vi "sub_main_joystick.vi"(8 "error in":errorcluster) -> (0 "error out":errorcluster)   [LabVIEW 2019]
uses:
  Ctrl/cmd_common.ctl
  Ctrl/sound-data.ctl
panel:
  out "error out check":errorcluster
  out "n":i32
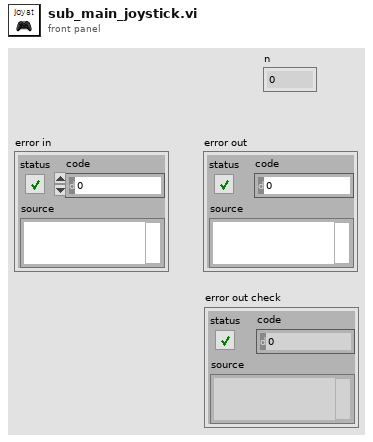
[diagram p1: front panel]
types:
  T1 = typedef "cmd_common.ctl" = enum16{"read", "write"}
  T2 = typedef "sound-data.ctl" = cluster{"FN":enum16{"check", "unlock", "engine", "warning", "msg", "music"}, "Data":variant}
  T3 = cluster{"axis info":cluster{"X axis":i32, "Y axis":i32, "Z axis":i32, "X axis rotation":i32, "Y axis rotation":i32, "Z axis rotation":i32, "U axis":i32, "V axis":i32}, "button info":cluster{"button 1":bool, "button 2":bool, "button 3":bool, "button 4":bool, "button 5":bool, "button 6":bool, "button 7":bool, "button 8":bool, "button 9":bool, "button 10":bool, "button 11":bool, "button 12":bool, "button 13":bool, "button 14":bool, "button 15":bool, "button 16":bool, "button 17":bool, "button 18":bool, "button 19":bool, "button 20":bool, "button 21":bool, "button 22":bool, "button 23":bool, "button 24":bool, "button 25":bool, "button 26":bool, "button 27":bool, "button 28":bool, "button 29":bool, "button 30":bool, "button 31":bool, "button 32":bool}, "direction info":cluster{"pov 1":i32, "pov 2":i32, "pov 3":i32, "pov 4":i32}}
  T4 = cluster{"button 1":bool, "button 2":bool, "button 3":bool, "button 4":bool, "button 5":bool, "button 6":bool, "button 7":bool, "button 8":bool, "button 9":bool, "button 10":bool, "button 11":bool, "button 12":bool, "button 13":bool, "button 14":bool, "button 15":bool, "button 16":bool, "button 17":bool, "button 18":bool, "button 19":bool, "button 20":bool, "button 21":bool, "button 22":bool, "button 23":bool, "button 24":bool, "button 25":bool, "button 26":bool, "button 27":bool, "button 28":bool, "button 29":bool, "button 30":bool, "button 31":bool, "button 32":bool}
  T5 = cluster{"pov 1":i32, "pov 2":i32, "pov 3":i32, "pov 4":i32}
  T6 = enum16{"check", "unlock", "engine", "warning", "msg", "music"}
  T7 = typedef "status.ctl" = u16
  T8 = cluster{"AGV":T7, "AGV Estop":T7, "Obstacle":T7, "Heading":T7, "Waypt":T7, "GNSS":T7, "VLP16":T7, "Cam":T7, "RPLidar":T7, "Joystick":T7, "IMU":T7}
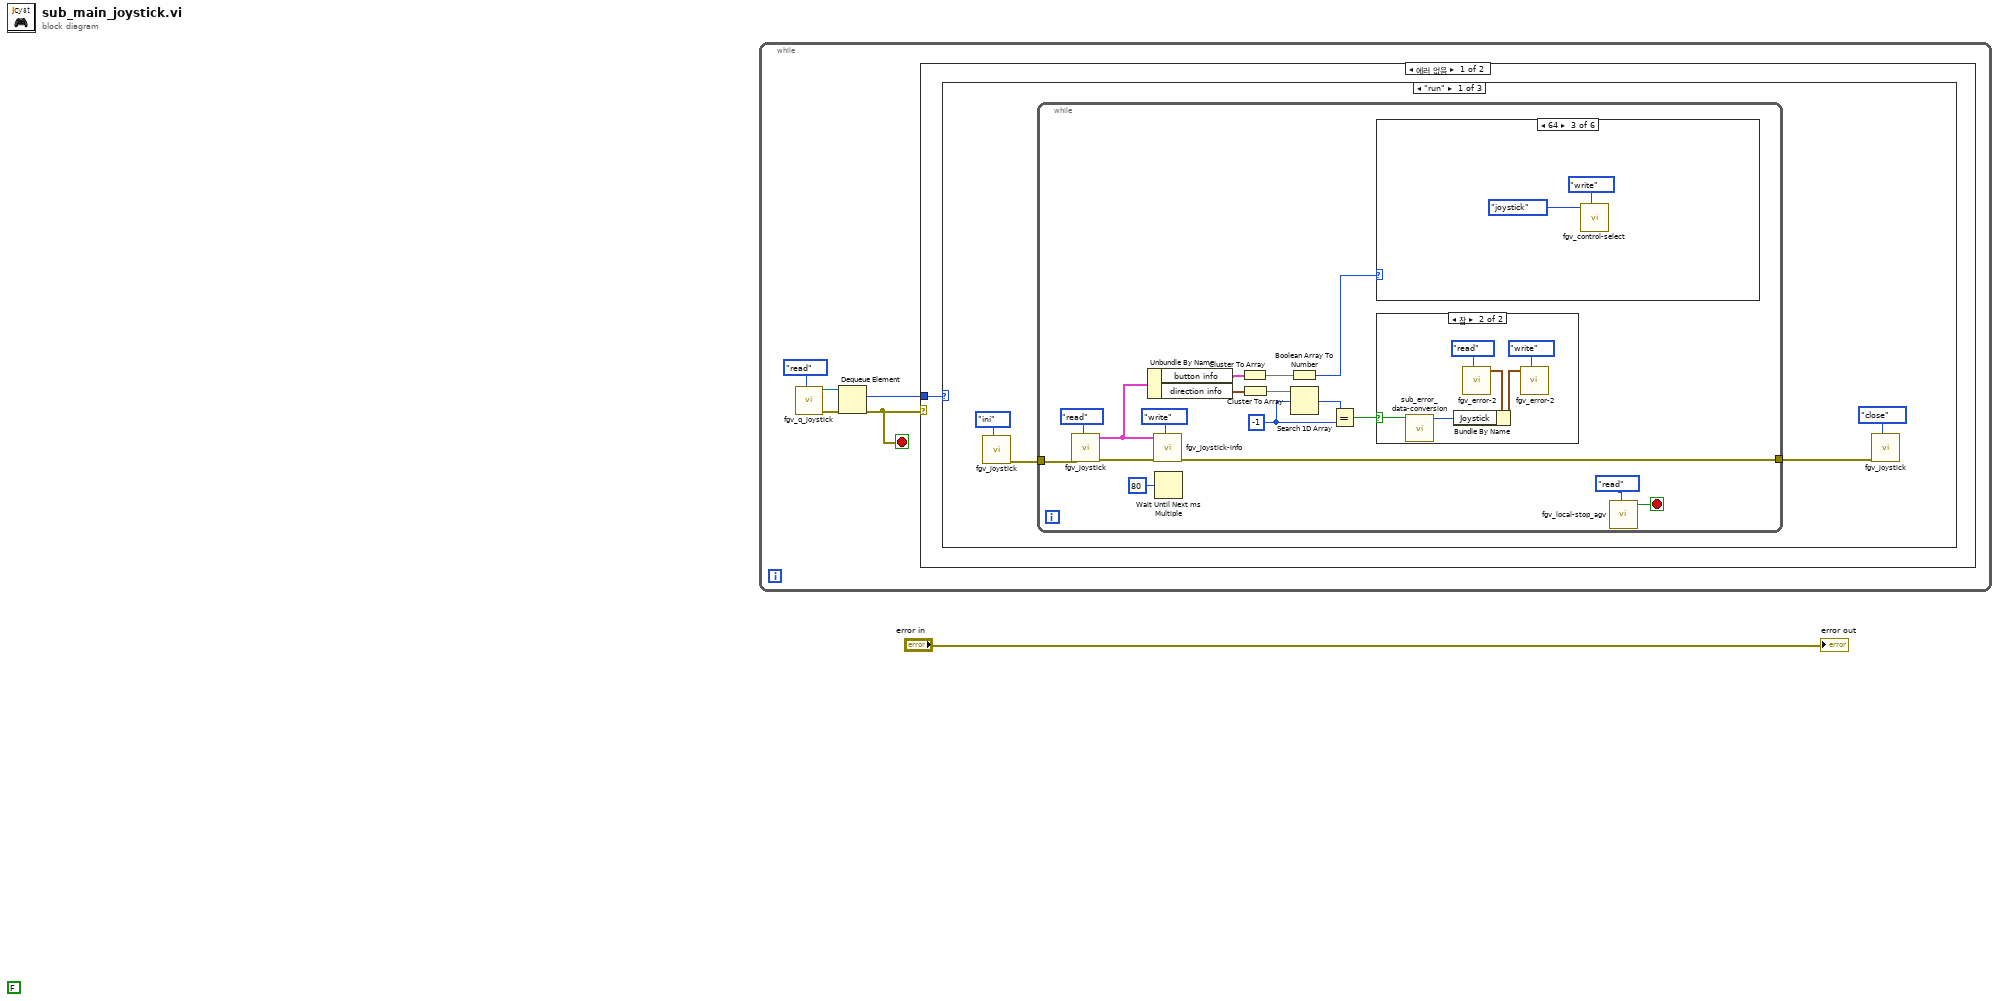
[diagram p0: block diagram]
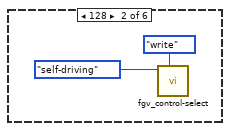
[diagram p3: hidden frame]
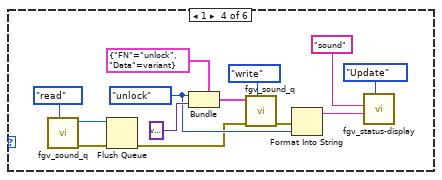
[diagram p4: hidden frame]
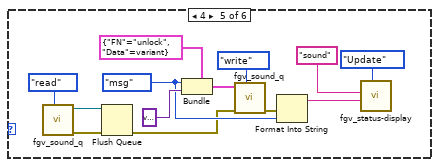
[diagram p5: hidden frame]
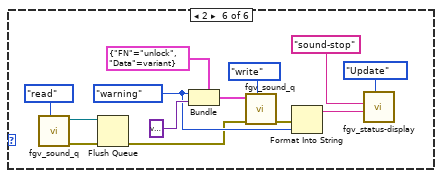
[diagram p6: hidden frame]
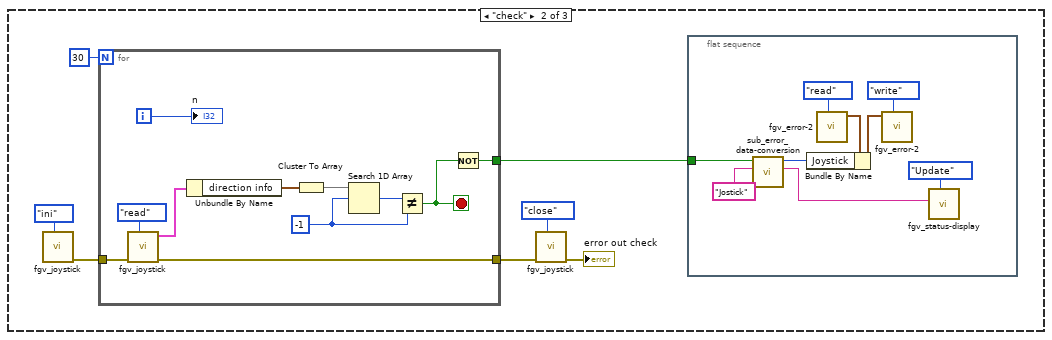
[diagram p8: hidden frame]
diagram:
  (unwired) FALSE
  n1 = while {
    stop <- w2 stop-if-true
    n2 = call "fgv_q_joystick.vi"("cmd"=enum16{"create", "write", "read", "close"}."read") -> ("error out"=w4:errorcluster, "queue out"=w5:refnum<queue>)  [unwired: 9 in]
    n3 = Dequeue Element(queue=w5, error in (no error)=w4) -> (element=w3:enum16{"run", "check", "stop"}, error out=w2:errorcluster)  [unwired: 1 in, 2 out]
    n4 = case shown="에러 없음" w2 {
      tunnel: w3 -> [w7 _]
      frame No Error {
        n5 = case shown="\"run\"" w7 {
          frame "run" {
            n6 = call "fgv_joystick.vi"("cmd"=enum16{"ini", "read", "close"}."ini") -> ("error out"=w9:errorcluster)  [unwired: 9 in, 1 out]
            n7 = while {
              tunnel: w9 -> [w23]
              tunnel: [w22] -> w8
              stop <- w27 stop-if-true
              w18 = -1 ("element")
              n8 = call "fgv_joystick.vi"("cmd"=enum16{"ini", "read", "close"}."read", "error in"=w23) -> ("error out"=w24:errorcluster, "joystick info-out"=w17:T3)  [unwired: 8 in]
              n9 = Unbundle By Name(w17) -> ("button info"=w14:T4, "direction info"=w21:T5)
              n10 = call "fgv_joystick-info.vi"("init"=enum16{"enable", "init", "read", "write"}."write", "error in"=w24, "joystick info-in"=w17) -> ("error out"=w22:errorcluster)  [unwired: 5 in, 3 out]
              n11 = Wait Until Next ms Multiple(millisecond multiple=u32 80 ("milliseconds to wait")) -> ()  [unwired: 1 out]
              n12 = Cluster To Array(cluster=w14) -> (array=w13:bool[])
              n13 = Cluster To Array(cluster=w21) -> (array=w20:i32[])
              n14 = Boolean Array To Number(Boolean array=w13) -> (number=w12:u32)
              n15 = Search 1D Array(1D array=w20, element=w18) -> (index of element=w19:i32)  [unwired: 1 in]
              n16 = Equal?(x=w19, y=w18) -> (x = y?=w15:bool)
              n17 = case shown="64" w12 {
                frame 0, Default {
                }
                frame 128 {
                  n18 = call "fgv_control-select.vi"("cmd"=cmd_common."write", "mode"=enum16{"joystick", "self-driving"}."self-driving") -> ()  [unwired: 9 in, 1 out]
                }
                frame 64 {
                  n19 = call "fgv_control-select.vi"("cmd"=cmd_common."write", "mode"=enum16{"joystick", "self-driving"}."joystick") -> ()  [unwired: 9 in, 1 out]
                }
                frame 1 {
                  w38 = T6."unlock" ("FN")
                  n20 = call "fgv_sound_q.vi"("cmd"=enum16{"create", "write", "read", "close"}."read") -> ("error out"=w35:errorcluster, "queue out"=w34:refnum<queue>)  [unwired: 9 in]
                  n21 = Flush Queue(queue=w34, error in (no error)=w35) -> (error out=w33:errorcluster)  [unwired: 2 out]
                  n22 = Bundle(cluster=T2 {"FN"=enum."unlock", "Data"=variant} ("data"), "FN"=w38, "Data"=variant) -> (w44:T2)
                  n23 = call "fgv_sound_q.vi"("cmd"=enum16{"create", "write", "read", "close"}."write", "error in"=w33, "data"=w44) -> ("error out"=w39:errorcluster)  [unwired: 7 in, 1 out]
                  n24 = Format Into String(error in=w39, w38) -> (resulting string=w37:string)  [unwired: 2 in, 1 out]
                  n25 = call "fgv_status-display.vi"("Mode"=enum16{"Initial", "Update", "Clear"}."Update", "detail"=w37, "title"="sound") -> ()  [unwired: 8 in, 1 out]
                }
                frame 4 {
                  w51 = T6."msg" ("FN")
                  n26 = call "fgv_sound_q.vi"("cmd"=enum16{"create", "write", "read", "close"}."read") -> ("error out"=w48:errorcluster, "queue out"=w47:refnum<queue>)  [unwired: 9 in]
                  n27 = Flush Queue(queue=w47, error in (no error)=w48) -> (error out=w46:errorcluster)  [unwired: 2 out]
                  n28 = Bundle(cluster=T2 {"FN"=enum."unlock", "Data"=variant} ("data"), "FN"=w51, "Data"=variant) -> (w57:T2)
                  n29 = call "fgv_sound_q.vi"("cmd"=enum16{"create", "write", "read", "close"}."write", "error in"=w46, "data"=w57) -> ("error out"=w52:errorcluster)  [unwired: 7 in, 1 out]
                  n30 = Format Into String(error in=w52, w51) -> (resulting string=w50:string)  [unwired: 2 in, 1 out]
                  n31 = call "fgv_status-display.vi"("Mode"=enum16{"Initial", "Update", "Clear"}."Update", "detail"=w50, "title"="sound") -> ()  [unwired: 8 in, 1 out]
                }
                frame 2 {
                  w64 = T6."warning" ("FN")
                  n32 = call "fgv_sound_q.vi"("cmd"=enum16{"create", "write", "read", "close"}."read") -> ("error out"=w61:errorcluster, "queue out"=w60:refnum<queue>)  [unwired: 9 in]
                  n33 = Flush Queue(queue=w60, error in (no error)=w61) -> (error out=w59:errorcluster)  [unwired: 2 out]
                  n34 = Bundle(cluster=T2 {"FN"=enum."unlock", "Data"=variant} ("data"), "FN"=w64, "Data"=variant) -> (w70:T2)
                  n35 = call "fgv_sound_q.vi"("cmd"=enum16{"create", "write", "read", "close"}."write", "error in"=w59, "data"=w70) -> ("error out"=w65:errorcluster)  [unwired: 7 in, 1 out]
                  n36 = Format Into String(error in=w65, w64) -> (resulting string=w63:string)  [unwired: 2 in, 1 out]
                  n37 = call "fgv_status-display.vi"("Mode"=enum16{"Initial", "Update", "Clear"}."Update", "detail"=w63, "title"="sound-stop") -> ()  [unwired: 8 in, 1 out]
                }
              }
              n38 = case shown="참" w15 {
                selector: w15 -> [_ w72]
                frame False {
                }
                frame True {
                  n39 = call "sub_error_data-conversion.vi"("error status"=w72) -> ("error conversion out"=w75:T7)  [unwired: 9 in, 1 out]
                  n40 = call "fgv_error-2.vi"("cmd"=enum16{"init", "read", "write"}."read") -> ("Error cluster out"=w74:T8)  [unwired: 9 in, 1 out]
                  n41 = Bundle By Name(cluster=w74, "Joystick"=w75) -> (w73:T8)
                  n42 = call "fgv_error-2.vi"("cmd"=enum16{"init", "read", "write"}."write", "Error cluster"=w73) -> ()  [unwired: 8 in, 2 out]
                }
              }
              n43 = call "fgv_local-stop_agv.vi"("cmd"=enum16{"ini", "read", "stop"}."read") -> ("stop status"=w27:bool)  [unwired: 10 in]
            }
            n44 = call "fgv_joystick.vi"("cmd"=enum16{"ini", "read", "close"}."close", "error in"=w8) -> ()  [unwired: 8 in, 2 out]
          }
          frame "check" {
            n45 = call "fgv_joystick.vi"("cmd"=enum16{"ini", "read", "close"}."ini") -> ("error out"=w83:errorcluster)  [unwired: 9 in, 1 out]
            n46 = for {
              N: 30 -> [_]
              tunnel: w83 -> [w104]
              tunnel: [w96] -> w80
              tunnel: [w94] -> w78
              i -> [w97]
              stop <- w95 stop-if-true
              w102 = -1 ("element")
              n47 = call "fgv_joystick.vi"("cmd"=enum16{"ini", "read", "close"}."read", "error in"=w104) -> ("error out"=w96:errorcluster, "joystick info-out"=w98:T3)  [unwired: 8 in]
              n48 = Unbundle By Name(w98) -> ("direction info"=w99:T5)
              n49 = Cluster To Array(cluster=w99) -> (array=w100:i32[])
              n50 = Search 1D Array(1D array=w100, element=w102) -> (index of element=w101:i32)  [unwired: 1 in]
              n51 = Not Equal?(x=w101, y=w102) -> (x != y?=w95:bool)
              n52 = Not(x=w95) -> (.not. x?=w94:bool)
              "n" <- w97
            }
            n53 = call "fgv_joystick.vi"("cmd"=enum16{"ini", "read", "close"}."close", "error in"=w80) -> ("error out"=→"error out check":errorcluster)  [unwired: 8 in, 1 out]
            n54 = flat-sequence {
              tunnel: w78 -> [w86]
              frame #0 {
                n55 = call "sub_error_data-conversion.vi"("name"="Jostick", "error status"=w86) -> ("check result string"=w87:string, "error conversion out"=w91:T7)  [unwired: 8 in]
                n56 = call "fgv_error-2.vi"("cmd"=enum16{"init", "read", "write"}."read") -> ("Error cluster out"=w92:T8)  [unwired: 9 in, 1 out]
                n57 = Bundle By Name(cluster=w92, "Joystick"=w91) -> (w93:T8)
                n58 = call "fgv_error-2.vi"("cmd"=enum16{"init", "read", "write"}."write", "Error cluster"=w93) -> ()  [unwired: 8 in, 2 out]
                n59 = call "fgv_status-display.vi"("Mode"=enum16{"Initial", "Update", "Clear"}."Update", "title"=w87) -> ()  [unwired: 9 in, 1 out]
              }
            }
          }
          frame "stop", Default {
          }
        }
      }
      frame Error {
      }
    }
  }
  "error out" <- "error in"
